vi "Int32Array Create.vi"(8 "error in (no error)":errorcluster, 11 "I32 array in":i32[](array[numeric])) -> (0 "error out":errorcluster, 3 "Int32Array DVR out":refnum<data-value>)   [LabVIEW 2012, in "MDSplus.lvlib"]
uses:
  <vilib>/MDSplus/Library/MDSplus.lvlib
  <vilib>/MDSplus/Classes/Data_Class/Array_Class/Int32Array_Class/Int32Array.lvclass
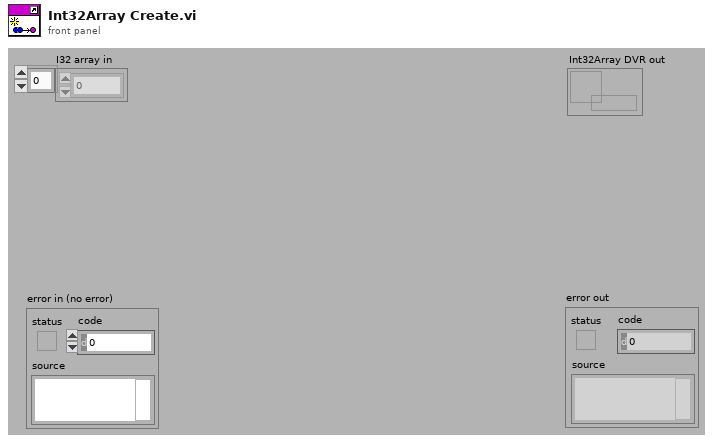
[diagram p1: front panel]
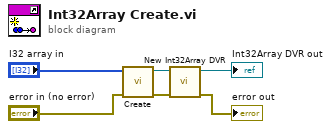
[diagram p0: block diagram]
diagram:
  n1 = call <vilib>:"Create.vi"("error in (no error)"="error in (no error)", "I32 array in"="I32 array in") -> ("error out"=w3:errorcluster, "Int32Array out"=w4:refnum<class "Int32Array.lvclass">)  [unwired: 8 in]
  n2 = call <vilib>:"New Int32Array DVR.vi"("error in (no error)"=w3, "Int32Array in"=w4) -> ("error out"=→"error out":errorcluster, "Int32Array DVR out"=→"Int32Array DVR out":refnum<data-value>)  [unwired: 8 in]
